vi "Obtain ID from Pool.vi"(8 "error in (no error)":errorcluster, 9 "timeout in ms (0)":i32 format="%d ms", 11 "ID Pool in":refnum<class "Pool ID.lvclass">) -> (0 "error out":errorcluster, 1 "timed out?":bool, 2 "id":i32, 3 "ID Pool out":refnum<class "Pool ID.lvclass">)   [LabVIEW 2017, in "Data Sharing Framework Core.lvlib" / "Data Sharing Framework Engine.lvlib" / "Pool ID.lvclass"]
uses:
  Pool ID.lvclass
  C:/github/data-sharing-framework/Source/Data Sharing Framework Core/Engine/Internal/Execution/Pool/Pool/Pool.lvclass
  Pool/Pool.lvclass/Pool.ctl
  Debug/Debug Flags FIFO/Debug Flags FIFO.lvclass/Debug Flags FIFO.ctl
  Pool/Get FIFO.vi
  Pool/Get Debug Flags.vi
  Debug/Debug Flags FIFO/Get Infinite Timeouts.vi
  Pool/Pool.lvclass
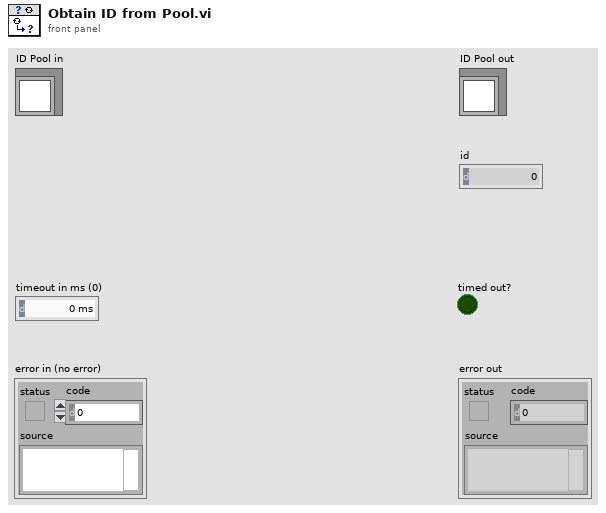
[diagram p1: front panel]
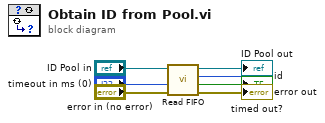
[diagram p0: block diagram]
diagram:
  n1 = call "Read FIFO.vi"("error in (no error)"="error in (no error)", "timeout in ms (0)"="timeout in ms (0)", "Pool in"="ID Pool in") -> ("error out"=→"error out":errorcluster, "timed out?"=→"timed out?":bool, "element"=→"id":i32, "Pool out"=→"ID Pool out":refnum<class "Pool ID.lvclass">)  [unwired: 5 in]
